vi "SimulateBPM.vi"() -> (3 "Simulated BPM":dbl[][](array[numeric]))   [LabVIEW 2012]
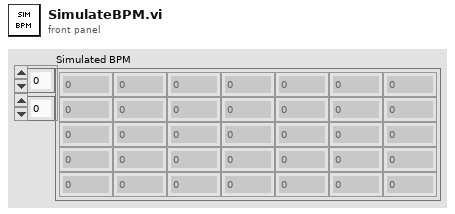
[diagram p1: front panel]
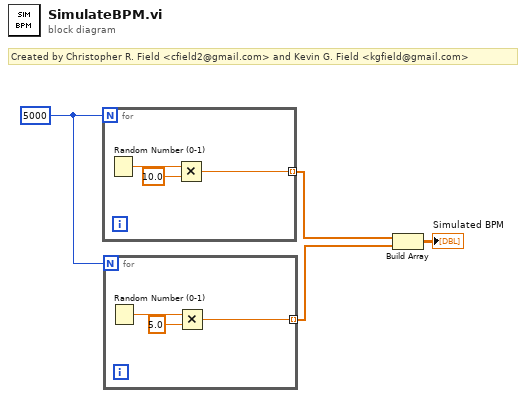
[diagram p0: block diagram]
diagram:
  w4 = 5000
  # "Created by Christopher R. Field <cfield2@gmail.com> and Kevin G. Field <kgfield@gmail.com>"
  n1 = for {
    N: w4 -> [_]
    tunnel: [w5] -> w3 mode=indexing
    n2 = Random Number (0-1)() -> (number: 0 to 1=w7:dbl)
    n3 = Multiply(x=w7, y=10.0) -> (x*y=w5:dbl)
  }
  n4 = for {
    N: w4 -> [_]
    tunnel: [w8] -> w2 mode=indexing
    n5 = Random Number (0-1)() -> (number: 0 to 1=w10:dbl)
    n6 = Multiply(x=w10, y=5.0) -> (x*y=w8:dbl)
  }
  n7 = Build Array(w3, w2) -> (→"Simulated BPM":dbl[][])
